vi "Find Supported Devices.vi"(8 "error in (no error)":errorcluster) -> (0 "error out":errorcluster, 2 "Supported Cameras":string[](array[string]), 3 "Camera Driver Paths":path[](array[path]))   [LabVIEW 2019]
uses:
  <vilib>/Utility/error.llb/Error Cluster From Error Code.vi
  <vilib>/ErrorRing/Error Ring.xnode
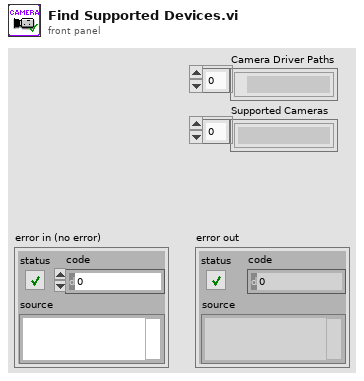
[diagram p1: front panel]
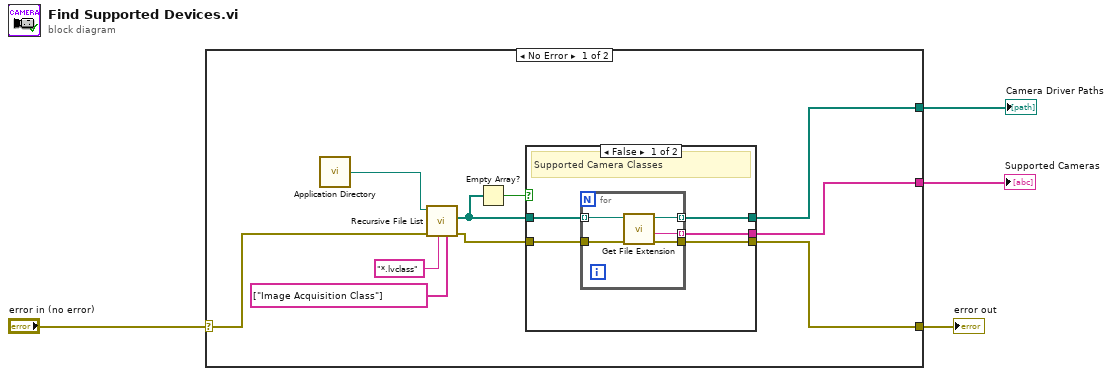
[diagram p0: block diagram]
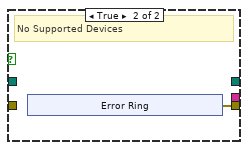
[diagram p2: hidden frame]
diagram:
  n1 = case shown="No Error" "error in (no error)" {
    selector: "error in (no error)" -> [w8 w31]
    tunnel: [w12 w31] -> w4
    tunnel: [w7 _] -> w2
    tunnel: [w6 _] -> w1
    frame No Error {
      n2 = call <vilib>:"Application Directory.vi"() -> ("Application Directory"=w5:path)
      n3 = call <vilib>:"Recursive File List.vi"("Folders to Exclude"=string[] ["Image Acquisition Class"], "pattern"="*.lvclass", "error in (no error)"=w8, "Folder Path"=w5) -> ("error out"=w9:errorcluster, "All Files in Dir"=w11:path[])  [unwired: 3 in, 3 out]
      n4 = Empty Array?(array=w11) -> (empty?=w10:bool)
      n5 = case shown="False" w10 {
        tunnel: [w19 w25] -> w12
        tunnel: w11 -> [w18 _]
        tunnel: w9 -> [w17 _]
        tunnel: [w16 _] -> w6
        tunnel: [w15 _] -> w7
        frame False {
          # "Supported Camera Classes"
          n6 = for {
            tunnel: [w24] -> w16 mode=indexing
            tunnel: w18 -> [w23] mode=indexing
            tunnel: [w22] -> w15 mode=indexing
            tunnel: [w21] -> w19
            tunnel: w17 -> [w20]
            n7 = call <vilib>:"Get File Extension.vi"("error in (no error)"=w20, "file"=w23) -> ("error out"=w21:errorcluster, "filename without extension"=w24:string, "dup file"=w22:path)  [unwired: 5 in, 2 out]
          }
        }
        frame True {
          # "No Supported Devices"
          n8 = xnode "Error Ring"() -> ("error out"=w25:errorcluster)
        }
      }
    }
    frame Error {
    }
  }
  "error out" <- w4
  "Camera Driver Paths" <- w2
  "Supported Cameras" <- w1
